vi "demo - first VI.vi"() -> ()   [LabVIEW 2024]
doc: "<B>Checks if Temperature exceeds threshold, in Celsius</B>"
panel:
  in  "Stop":bool
  out "Waveform Chart":dbl(graph)
  out "Alarm":bool
  in  "Threshold":dbl
  in  "Current Temperature":dbl
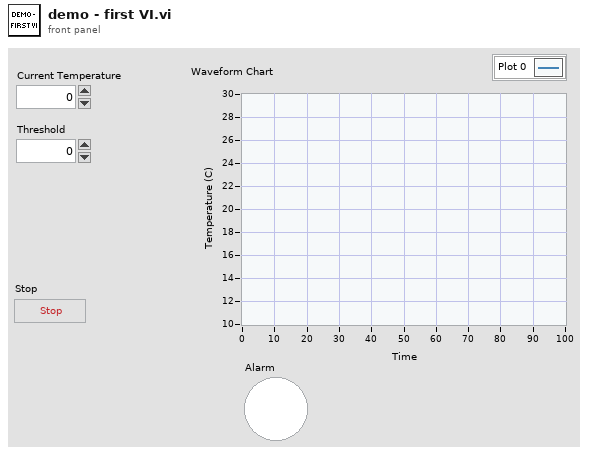
[diagram p1: front panel]
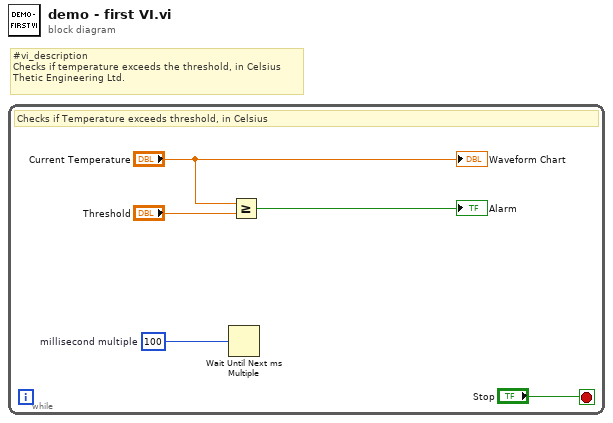
[diagram p0: block diagram]
diagram:
  # "#vi_description \nChecks if temperature exceeds the threshold, in Celsius\nThetic Engineering Ltd."
  n1 = while {
    stop <- "Stop" stop-if-true
    w1 = u32 100  # millisecond multiple
    # "Checks if Temperature exceeds threshold, in Celsius"
    n2 = Wait Until Next ms Multiple(millisecond multiple=w1) -> ()  [unwired: 1 out]
    n3 = Greater Or Equal?(x="Current Temperature", y="Threshold") -> (x >= y?=→"Alarm":bool)
    "Waveform Chart" <- "Current Temperature"
  }
